vi "start.vi"() -> ()   [LabVIEW 2014]
panel:
  out "系统启动中":u8(slide) scale=0.0..5.0
  out "Current Status 2":string
  # "Version: C.1.0\n--\n南京天创智能"
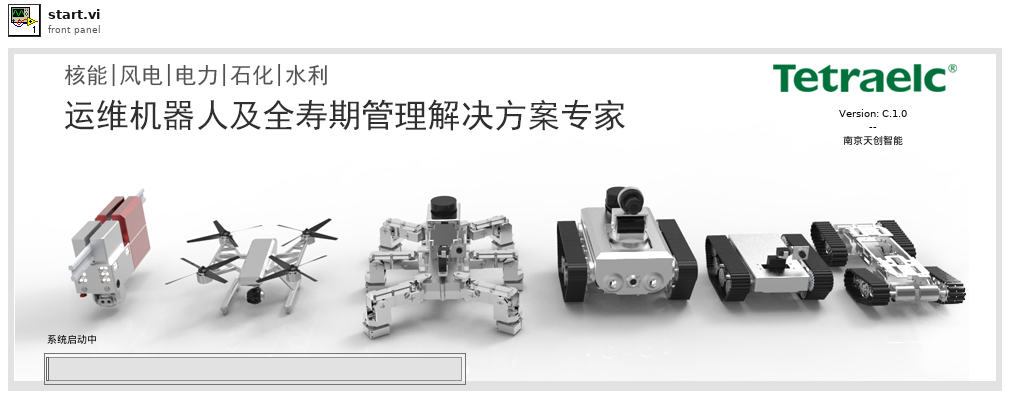
[diagram p1: front panel]
types:
  T1 = enum32{"Invalid", "Standard", "Closed", "Hidden", "Minimized", "Maximized"}
  T2 = enum32{"invalid app kind", "Development System", "Run Time System", "Student Edition", "Embedded LabVIEW", "Evaluation", "Custom"}
  T3 = enum32{"Bad", "Idle", "Run top level", "Running"}
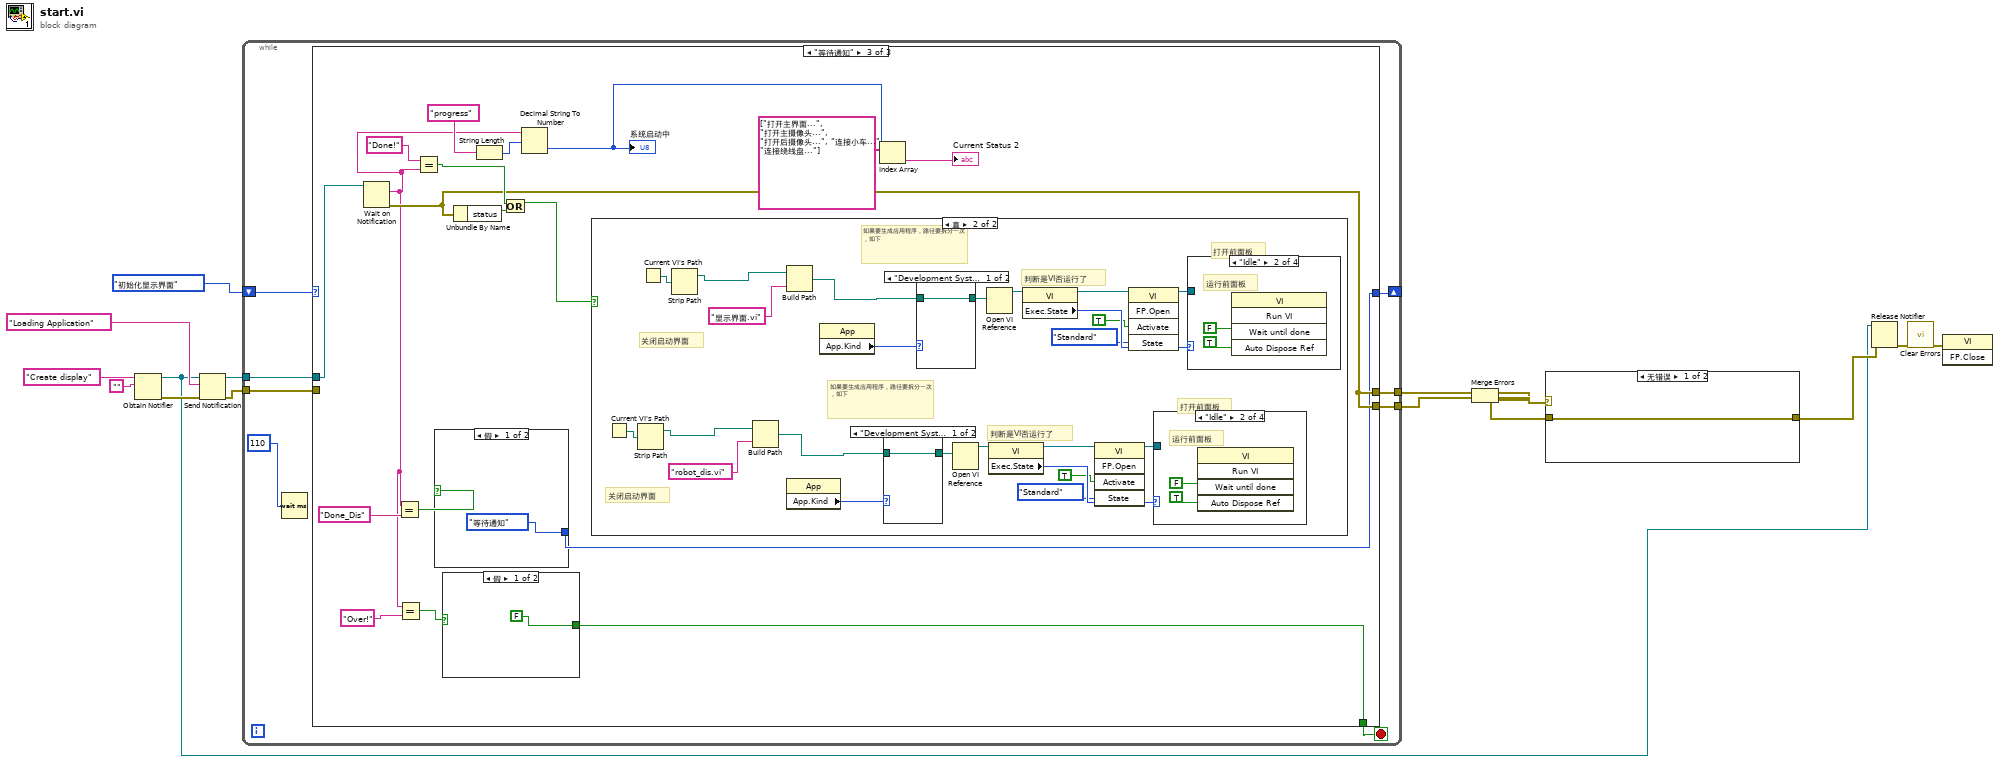
[diagram p0: block diagram]
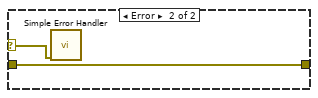
[diagram p2: hidden frame]
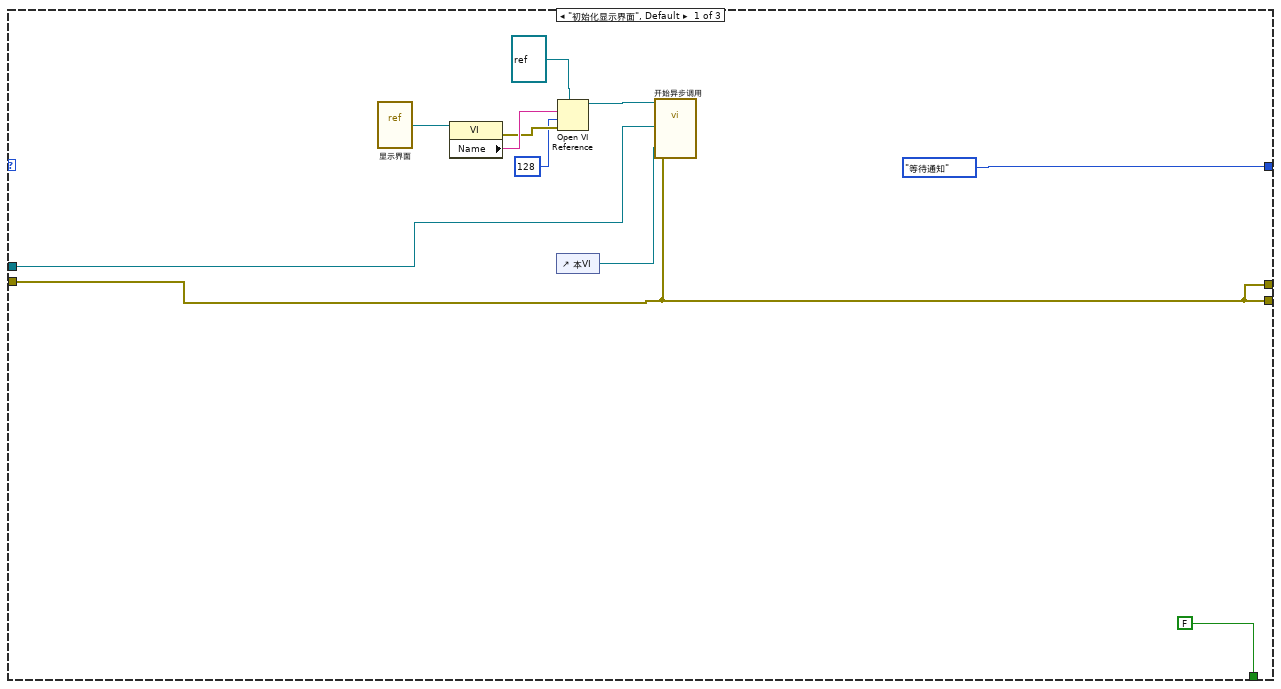
[diagram p3: hidden frame]
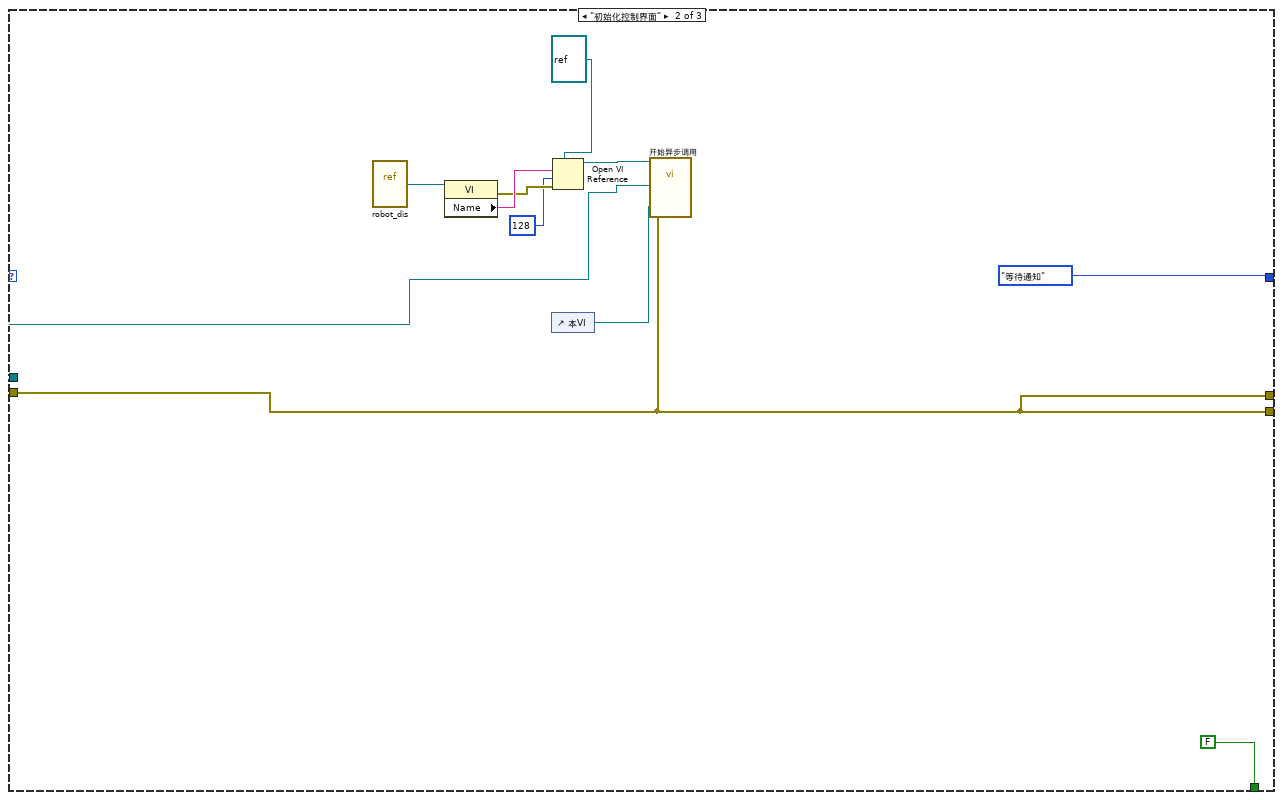
[diagram p4: hidden frame]
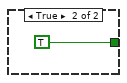
[diagram p5: hidden frame]
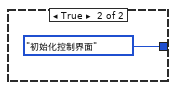
[diagram p6: hidden frame]
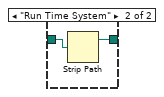
[diagram p8: hidden frame]
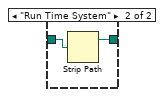
[diagram p12: hidden frame]
diagram:
  n1 = Obtain Notifier(name (unnamed)="Create display" ("名称（未命名）"), notification data type="") -> (notifier out=w1:refnum<notifier>, error out=w12:errorcluster)  [unwired: 2 in, 1 out]
  n2 = Send Notification(notification="Loading Application", notifier=w1, error in (no error)=w12) -> (notifier out=w10:refnum<notifier>, error out=w9:errorcluster)
  n3 = while {
    tunnel: w10 -> [w22]
    tunnel: w9 -> [w21]
    shift-right: [w19] -> _
    shift-left: enum16{"等待通知", "初始化显示界面", "初始化控制界面"}."初始化显示界面" -> [w20]
    tunnel: [w18] -> w3
    tunnel: [w17] -> w2
    stop <- w16 stop-if-true
    n4 = Wait (ms)(milliseconds to wait=u32 110 ("毫秒计时值")) -> ()  [unwired: 1 out]
    n5 = case shown="\"等待通知\"" w20 {
      tunnel: w22 -> [w32 w43 w54]
      tunnel: w21 -> [w31 w42 _]
      tunnel: [enum16{"等待通知", "初始化显示界面", "初始化控制界面"}."等待通知" enum16{"等待通知", "初始化显示界面", "初始化控制界面"}."等待通知" w49] -> w19
      tunnel: [w31 w42 w52] -> w18
      tunnel: [w31 w42 w52] -> w17
      tunnel: [FALSE FALSE w45] -> w16
      frame "初始化显示界面", Default {
        n6 = vi-ref "显示界面.vi"() -> (w24:refnum<vi>)
        n7 = property class="VI"(reference=w24) -> (error out=w29:errorcluster, "Name"=w30:string)  [unwired: 1 in, 1 out]
        n8 = control-ref of="本VI"() -> (w25:refnum<vi>)
        n9 = Open VI Reference(type specifier VI Refnum (for type only)=refnum<vi> refnum, vi path=w30, options=128 ("选项"), error in (no error)=w29) -> (vi reference=w26:refnum<vi>)  [unwired: 2 in, 1 out]
        n10 = call-by-ref "开始异步调用"(reference=w26, "VI引用句柄"=w25, "error in (no error)"=w31, "状态通知器"=w32) -> ()  [unwired: 1 in, 3 out]
      }
      frame "初始化控制界面" {
        n11 = vi-ref "robot_dis.vi"() -> (w41:refnum<vi>)
        n12 = property class="VI"(reference=w41) -> (error out=w39:errorcluster, "Name"=w40:string)  [unwired: 1 in, 1 out]
        n13 = control-ref of="本VI"() -> (w35:refnum<vi>)
        n14 = Open VI Reference(type specifier VI Refnum (for type only)=refnum<vi> refnum, vi path=w40, options=128 ("选项"), error in (no error)=w39) -> (vi reference=w36:refnum<vi>)  [unwired: 2 in, 1 out]
        n15 = call-by-ref "开始异步调用"(reference=w36, "VI引用句柄"=w35, "error in (no error)"=w42, "状态通知器"=w43) -> ()  [unwired: 1 in, 3 out]
      }
      frame "等待通知" {
        n16 = Wait on Notification(notifier=w54) -> (notification=w48:string, error out=w52:errorcluster)  [unwired: 3 in, 2 out]
        n17 = Equal?(x=w48, y="Done_Dis" ("notification")) -> (x = y?=w50:bool)
        n18 = Equal?(x=w48, y="Over!" ("notification")) -> (x = y?=w46:bool)
        n19 = Equal?(x="Done!" ("notification"), y=w48) -> (x = y?=w55:bool)
        n20 = case shown="假" w50 {
          tunnel: [enum16{"等待通知", "初始化显示界面", "初始化控制界面"}."等待通知" enum16{"等待通知", "初始化显示界面", "初始化控制界面"}."初始化控制界面"] -> w49
          frame False {
          }
          frame True {
          }
        }
        n21 = case shown="假" w46 {
          tunnel: [FALSE TRUE] -> w45
          frame False {
          }
          frame True {
          }
        }
        n22 = Unbundle By Name(w52) -> ("status"=w61:bool)
        n23 = String Length(string="progress" ("搜索字符串/字符(-)")) -> (length=w59:i32)
        n24 = Or(x=w55, y=w61) -> (x .or. y?=w53:bool)
        n25 = Decimal String To Number(string=w48, offset=w59) -> (number=w56:i32)  [unwired: 1 in, 1 out]
        "系统启动中" <- w56
        n26 = case shown="真" w53 {
          frame False {
          }
          frame True {
            # "如果要生成应用程序，路径要拆分一次，如下"
            # "判断是VI否运行了"
            # "打开前面板"
            # "关闭启动界面"
            # "如果要生成应用程序，路径要拆分一次，如下"
            # "判断是VI否运行了"
            # "打开前面板"
            # "关闭启动界面"
            n27 = Current VI's Path() -> (path=w77:path)
            n28 = Strip Path(path=w77) -> (stripped path=w67:path)  [unwired: 1 out]
            n29 = Current VI's Path() -> (path=w89:path)
            n30 = Strip Path(path=w89) -> (stripped path=w79:path)  [unwired: 1 out]
            n31 = Build Path(base path=w67, name or relative path="robot_dis.vi" ("名称或相对路径")) -> (appended path=w68:path)
            n32 = Build Path(base path=w79, name or relative path="显示界面.vi" ("名称或相对路径")) -> (appended path=w80:path)
            n33 = property class="App"() -> ("App.Kind"=w70:T2)  [unwired: 2 in, 2 out]
            n34 = property class="App"() -> ("App.Kind"=w82:T2)  [unwired: 2 in, 2 out]
            n35 = case shown="\"Development System\", 默认" w70 {
              tunnel: [w91 w92] -> w69
              tunnel: w68 -> [w91 w93]
              frame "Development System", Default {
              }
              frame "Run Time System" {
                n36 = Strip Path(path=w93) -> (stripped path=w92:path)  [unwired: 1 out]
              }
            }
            n37 = case shown="\"Development System\", 默认" w82 {
              tunnel: [w96 w97] -> w81
              tunnel: w80 -> [w96 w98]
              frame "Development System", Default {
              }
              frame "Run Time System" {
                n38 = Strip Path(path=w98) -> (stripped path=w97:path)  [unwired: 1 out]
              }
            }
            n39 = Open VI Reference(vi path=w69) -> (vi reference=w76:refnum<vi>)  [unwired: 5 in, 1 out]
            n40 = Open VI Reference(vi path=w81) -> (vi reference=w88:refnum<vi>)  [unwired: 5 in, 1 out]
            n41 = property class="VI"(reference=w76) -> (reference out=w72:refnum<vi>, "Exec.State"=w75:T3)  [unwired: 1 in, 1 out]
            n42 = property class="VI"(reference=w88) -> (reference out=w84:refnum<vi>, "Exec.State"=w87:T3)  [unwired: 1 in, 1 out]
            n43 = invoke class="VI" method="FP.Open"(reference=w72, "Activate"=TRUE ("Activate?"), "State"=T1."Standard") -> (reference out=w71:refnum<vi>)  [unwired: 2 in, 4 out]
            n44 = invoke class="VI" method="FP.Open"(reference=w84, "Activate"=TRUE ("Activate?"), "State"=T1."Standard") -> (reference out=w83:refnum<vi>)  [unwired: 2 in, 4 out]
            n45 = case shown="\"Idle\"" w75 {
              tunnel: w71 -> [_ _ _ _]
              frame "Bad", Default {
              }
              frame "Idle" {
                # "运行前面板"
                n46 = invoke class="VI" method="Run VI"("Wait until done"=FALSE ("结束前等待"), "Auto Dispose Ref"=TRUE ("自动销毁引用")) -> ()  [unwired: 3 in, 5 out]
              }
              frame "Run top level" {
              }
              frame "Running" {
              }
            }
            n47 = case shown="\"Idle\"" w87 {
              tunnel: w83 -> [_ _ _ _]
              frame "Bad", Default {
              }
              frame "Idle" {
                # "运行前面板"
                n48 = invoke class="VI" method="Run VI"("Wait until done"=FALSE ("结束前等待"), "Auto Dispose Ref"=TRUE ("自动销毁引用")) -> ()  [unwired: 3 in, 5 out]
              }
              frame "Run top level" {
              }
              frame "Running" {
              }
            }
          }
        }
        n49 = Index Array(array=string[] ["打开主界面...", "打开主摄像头...", "打开后摄像头...", "连接小车...", "连接绕线盘..."], index=w56) -> (element=→"Current Status 2":string)
      }
    }
  }
  n50 = Merge Errors(w2, w3) -> (w4:errorcluster)
  n51 = case shown="无错误" w2 {
    tunnel: [w101 w102] -> w5
    tunnel: w4 -> [w101 w102]
    selector: w2 -> [_ w103]
    frame No Error {
    }
    frame Error {
      n52 = call <vilib>:"Simple Error Handler.vi"("error in (no error)"=w103) -> ()  [unwired: 4 in, 5 out]
    }
  }
  n53 = Release Notifier(notifier=w1, error in (no error)=w5) -> (error out=w7:errorcluster)  [unwired: 1 in, 2 out]
  n54 = call <vilib>:"Clear Errors.vi"("error in (no error)"=w7) -> ("error out"=w6:errorcluster)  [unwired: 5 in, 1 out]
  n55 = invoke class="VI" method="FP.Close"(error in=w6) -> ()  [unwired: 2 in, 3 out]
